vi "SweepCtrlStepCal_DP_ver2.0.vi"(0 "output cluster":T1={"Main Sweep"=0, "Steps Config:"={"total points:"=0, "Step Delay (s)"=0.0, "Ini Delay (s)"=0.0, "# of steps:"=0}, "Temperature Control (ITC 503):"={"GPIB ADR"=0, "Change Heater?"={"Heater?"=FALSE, "Heater"=0}, "Change Temp?"={"Change T?"=FALSE, "Set T (K)"=0.0}, "Cluster"={"Heat Auto?"=FALSE, "Manual Heat?"=FALSE, "Heater (%)"=0.0}, "Change PID?"={"Change PID?"=FALSE, "P"=0.0, "I"=0.0, "D"=0.0}, "Change Para?"=FALSE, "Sensor"=1}, "Temperature Control (LS 340):"={"GPIB ADR"=0, "From (K)"=0.0, "To (K)"=0.0, "Rate (K/min)"=0.0, "Delta T (0.08K)"=0.0, "Temp. Header"="", "T Display Control"={"Ch B"=FALSE, "Ch C"=FALSE, "Ch D"=FALSE}}, "Magnet Control (IPS 120-10)"={"Action"=0, "Standby (s)"=0.0, "Heater on (s)"=0.0, "Sweep Setup "=[], "GPIB ADR"=0, "Change Para?"=FALSE}, "Keithley 6221 :"=[], "Measuring Instruments : "=[], "Lock-In SR7265 :"=[], "Deascription of \nthis measurement"="", "Instruments Config:"=[], "LS372 Bridge : 2"=[{"GPIB"=0, "Excitation"=0, "Autorange?"=FALSE, "Range"=0, "Current"=0, "Voltage"=0, "DataHeader"="Rx;Ry"}], "Magnet Control (CS4) 2"={"Action"=1, "Standby (s)"=0.0, "Heater on (s)"=300.0, "Sweep Setup "=[], "GPIB ADR"=0, "Change Para?"=FALSE}} {"Magnet Control (CS4) 2"."GPIB ADR" items=["None"=0, "25"=25]; "Magnet Control (CS4) 2"."Sweep Setup"."Rate in Range (T/min)" min=0.001 max=0.5 step=0.001; "Magnet Control (CS4) 2"."Sweep Setup"."Hold(min)" min=0.0; "Magnet Control (CS4) 2"."Sweep Setup"."Set Point (T)" min=-9.0 max=9.0 step=0.001; "Magnet Control (CS4) 2"."Action" items=["Up", "Down", "Pause", "Zero"]; "LS372 Bridge : 2"."Voltage" items=["2.00 uV"=1, "6.32 uV"=2, "20.0 uV"=3, "63.2 uV"=4, "200 uV"=5, "632 uV"=6, "2.0 mV"=7, "6.32 mV"=8]; "LS372 Bridge : 2"."Current" items=["1.00 pA"=1, "3.16 pA"=2, "10.0 pA"=3, "31.6 pA"=4, "100 pA"=5, "316 pA"=6, "1.00 nA"=7, "3.16 nA"=8, "10 nA"=9, "31.6 nA"=10, "100 nA"=11, "316 nA"=12, "1.00 uA"=13, "3.16 uA"=14, "10.0 uA"=15, "31.6 uA"=16, "100 uA"=17, "316 uA"=18, "1.00 mA"=19, "3.16 mA"=20, "10.0 mA"=21, "31.6 mA"=22]; "LS372 Bridge : 2"."Range" items=["2.0 m"=1, "6.32 m"=2, "20.0 m"=3, "63.2 m"=4, "200 m"=5, "632 m"=6, "2.00"=7, "6.32"=8, "20.0"=9, "63.2"=10, "200"=11, "632"=12, "2.00 k"=13, "6.32 k"=14, "20.0 k"=15, "63.2 k"=16, "200 k"=17, "632 k"=18, "2.00 M"=19, "6.32 M"=20, "20.0 M"=21, "63.2 M"=22]; "LS372 Bridge : 2"."Excitation" items=["Voltage", "Current"]; "LS372 Bridge : 2"."GPIB" items=["None"=0, "9"=9]; "Main Sweep" items=["Time", "DC Current", "Delta Current", "Pulse Delta Current", "Sine Current", "Lock-in Vosc"]; "Temperature Control (ITC 503):"."Sensor" items=["T2", "T3"]; "Magnet Control (IPS 120-10)"."Action" items=["Hold", "To Set point", "To Zero", "Clamp"]; "Keithley 6221 :"."Sweep Mode" items=["Linear", "Log", "Exp", "Inverse", "Manual"]}) -> (1 "Stay duration pts":dbl[](array[numeric]), 2 "2D Array of DC Source or Lock-In Ctrl Run Cluster":cluster{"GPIB ADR":u16, "DC St. Pt.":dbl}[][](array[cluster]))   [LabVIEW 2012]
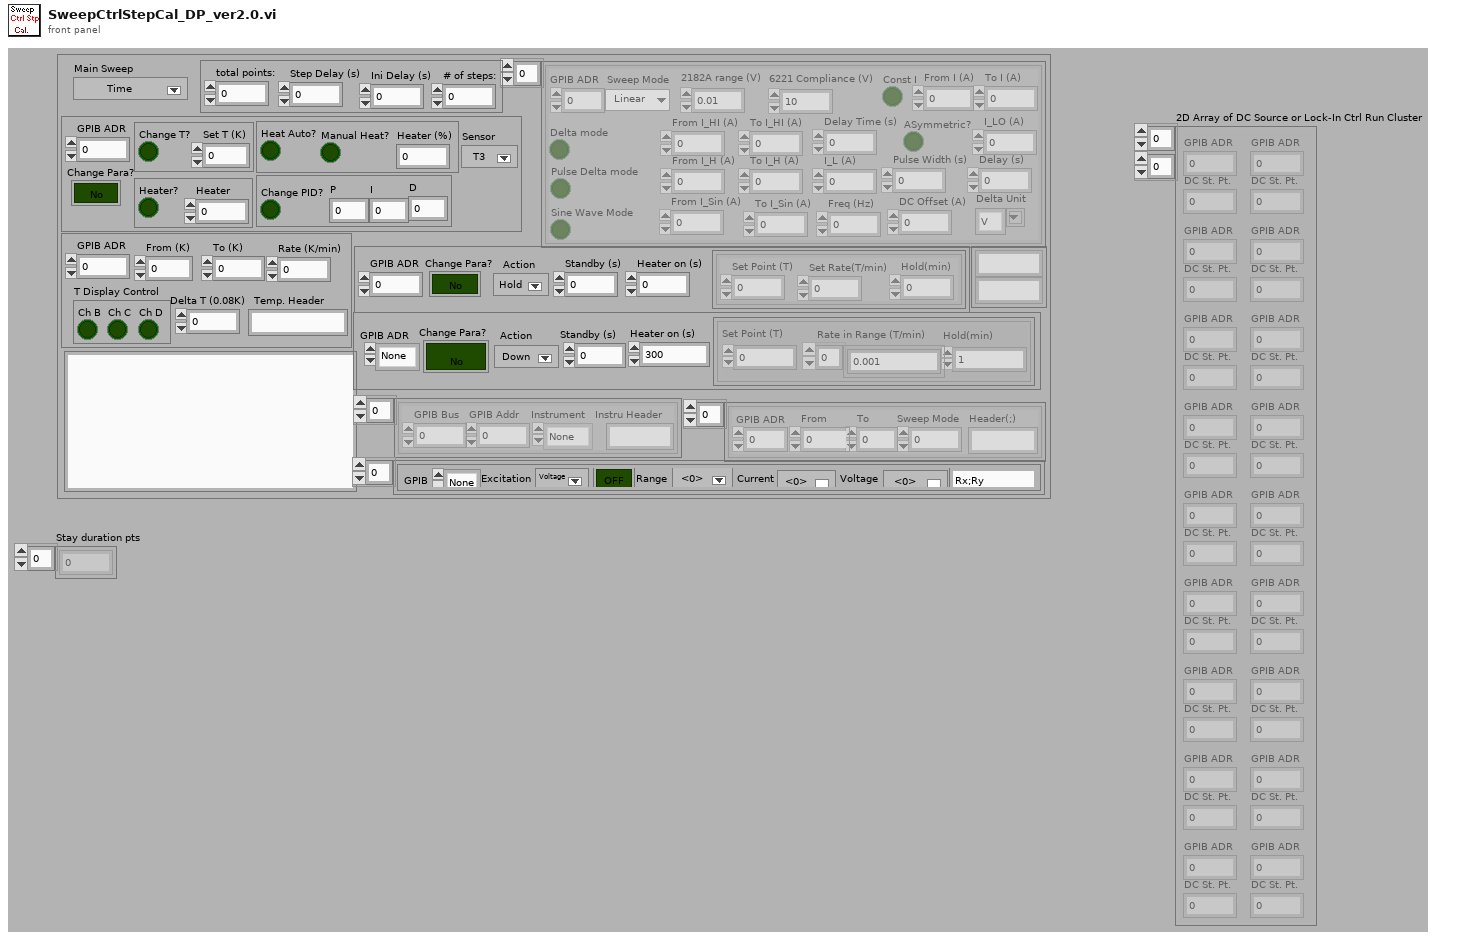
[diagram p1: front panel]
types:
  T1 = cluster{"Main Sweep":u8, "Steps Config:":cluster{"total points:":u32, "Step Delay (s)":dbl, "Ini Delay (s)":dbl, "# of steps:":u32}, "Temperature Control (ITC 503):":cluster{"GPIB ADR":u16, "Change Heater?":cluster{"Heater?":bool, "Heater":u8}, "Change Temp?":cluster{"Change T?":bool, "Set T (K)":dbl}, "Cluster":cluster{"Heat Auto?":bool, "Manual Heat?":bool, "Heater (%)":dbl}, "Change PID?":cluster{"Change PID?":bool, "P":dbl, "I":dbl, "D":dbl}, "Change Para?":bool, "Sensor":u16}, "Temperature Control (LS 340):":cluster{"GPIB ADR":u16, "From (K)":dbl, "To (K)":dbl, "Rate (K/min)":dbl, "Delta T (0.08K)":dbl, "Temp. Header":string, "T Display Control":cluster{"Ch B":bool, "Ch C":bool, "Ch D":bool}}, "Magnet Control (IPS 120-10)":cluster{"Action":u16, "Standby (s)":dbl, "Heater on (s)":dbl, "Sweep Setup ":cluster{"Set Point (T)":dbl, "Set Rate(T/min)":dbl, "Hold(min)":dbl}[], "GPIB ADR":u16, "Change Para?":bool}, "Keithley 6221 :":cluster{"Delta mode":bool, "Const I":bool, "Pulse Delta mode":bool, "Sine Wave Mode":bool, "From I_HI (A)":dbl, "From I (A)":dbl, "I_LO (A)":dbl, "From I_H (A)":dbl, "I_L (A)":dbl, "Freq (Hz)":dbl, "From I_Sin (A)":dbl, "DC Offset (A)":dbl, "Delay Time (s)":dbl, "Pulse Width (s)":dbl, "Delay (s)":dbl, "To I (A)":dbl, "ASymmetric?":bool, "To I_HI (A)":dbl, "To I_H (A)":dbl, "To I_Sin (A)":dbl, "GPIB ADR":u16, "Sweep Mode":u8, "Delta Unit":string, "2182A range (V)":dbl, "6221 Compliance (V)":dbl}[], "Measuring Instruments : ":cluster{"GPIB Bus":dbl, "GPIB Addr":dbl, "Instrument":enum16{"None", "HP34401DMM", "Lockin 7265", "HP3456/7A", "HP3478A", "HP3325FG", "Keithley2182A"}, "Instru Header":string}[], "Lock-In SR7265 :":cluster{"GPIB ADR":u16, "From":dbl, "To":dbl, "Header(;)":string, "Sweep Mode":u8}[], "Deascription of \nthis measurement":string, "Instruments Config:":string[][], "LS372 Bridge : 2":cluster{"GPIB":u16, "Excitation":u16, "Autorange?":bool, "Range":u16, "Current":u16, "Voltage":u16, "DataHeader":string}[], "Magnet Control (CS4) 2":cluster{"Action":u16, "Standby (s)":dbl, "Heater on (s)":dbl, "Sweep Setup ":cluster{"Set Point (T)":dbl, "Hold(min)":dbl, "Rate in Range (T/min)":dbl[]}[], "GPIB ADR":u16, "Change Para?":bool}}
  T2 = cluster{"total points:":u32, "Step Delay (s)":dbl, "Ini Delay (s)":dbl, "# of steps:":u32}
  T3 = cluster{"GPIB ADR":u16, "From":dbl, "To":dbl, "Header(;)":string, "Sweep Mode":u8}[]
  T4 = cluster{"Delta mode":bool, "Const I":bool, "Pulse Delta mode":bool, "Sine Wave Mode":bool, "From I_HI (A)":dbl, "From I (A)":dbl, "I_LO (A)":dbl, "From I_H (A)":dbl, "I_L (A)":dbl, "Freq (Hz)":dbl, "From I_Sin (A)":dbl, "DC Offset (A)":dbl, "Delay Time (s)":dbl, "Pulse Width (s)":dbl, "Delay (s)":dbl, "To I (A)":dbl, "ASymmetric?":bool, "To I_HI (A)":dbl, "To I_H (A)":dbl, "To I_Sin (A)":dbl, "GPIB ADR":u16, "Sweep Mode":u8, "Delta Unit":string, "2182A range (V)":dbl, "6221 Compliance (V)":dbl}[]
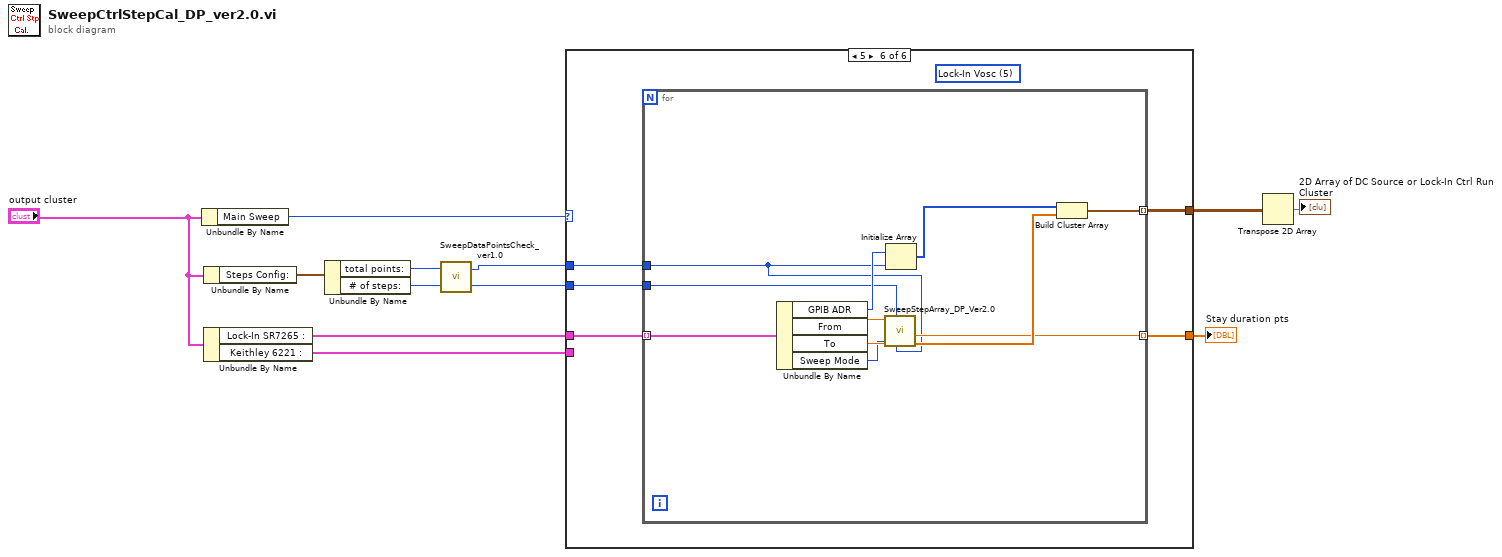
[diagram p0: block diagram]
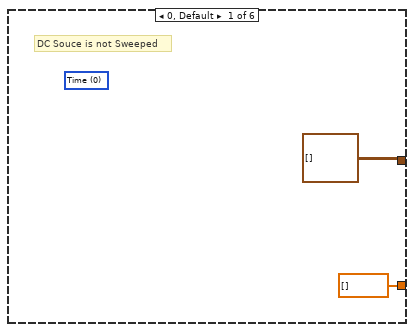
[diagram p2: hidden frame]
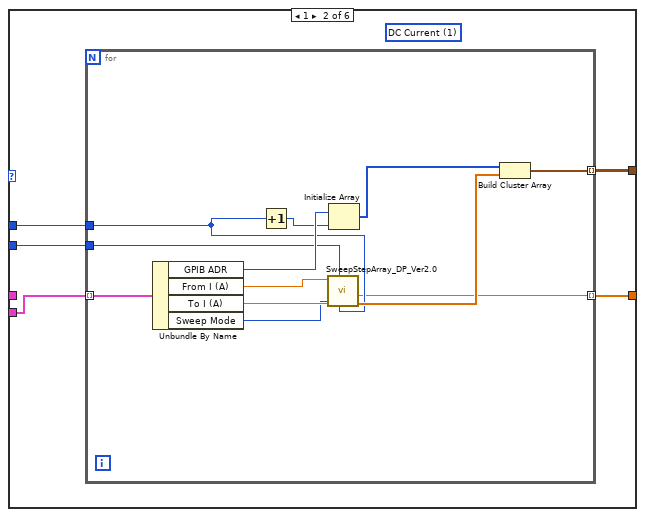
[diagram p3: hidden frame]
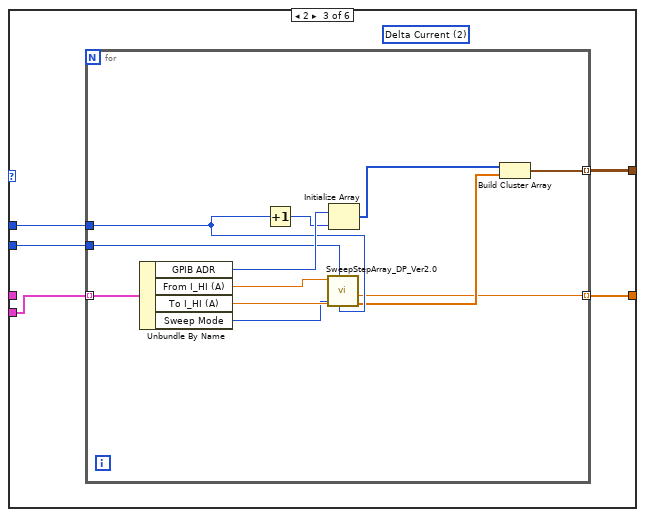
[diagram p4: hidden frame]
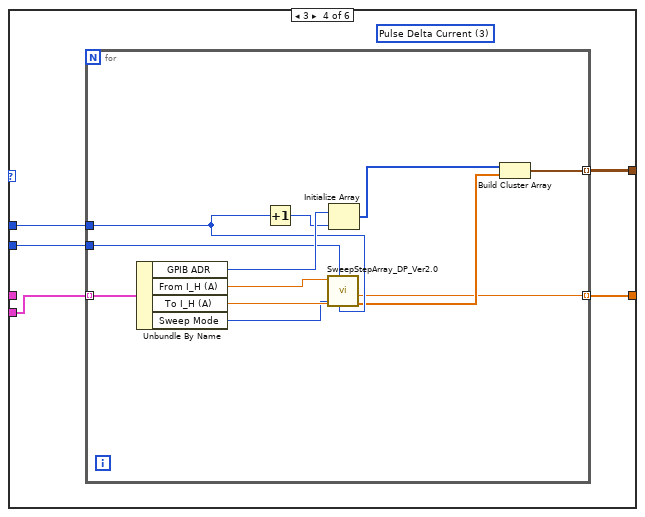
[diagram p5: hidden frame]
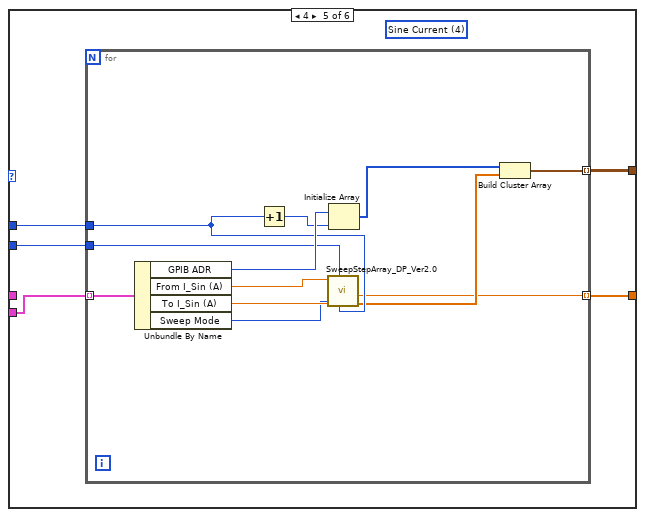
[diagram p6: hidden frame]
diagram:
  n1 = Unbundle By Name("output cluster") -> ("Main Sweep"=w10:u8)
  n2 = Unbundle By Name("output cluster") -> ("Steps Config:"=w9:T2)
  n3 = Unbundle By Name("output cluster") -> ("Lock-In SR7265 :"=w11:T3, "Keithley 6221 :"=w8:T4)
  n4 = Unbundle By Name(w9) -> ("total points:"=w7:u32, "# of steps:"=w6:u32)
  n5 = call "SweepDataPointsCheck_ver1.0.vi"("Input # of sweep steps:"=w6, "Input # of total points:"=w7) -> ("Output # of sweep steps:"=w2:u32, "Output # of total points:"=w5:u32)
  n6 = case shown="5" w10 {
    tunnel: [cluster{"GPIB ADR":u16, "V Start":dbl}[][] [] ("array of clusters") w19 w36 w53 w70 w87] -> w4
    tunnel: w11 -> [_ _ _ _ _ w86]
    tunnel: w5 -> [_ w18 w35 w52 w69 w85]
    tunnel: w2 -> [_ w17 w34 w51 w68 w84]
    tunnel: w8 -> [_ w16 w33 w50 w67 _]
    tunnel: [dbl[] [] w15 w32 w49 w66 w83] -> w3
    frame 0, Default {
      (unwired) u8 0 items=["Time", "DC Current", "Delta Current", "Pulse Delta Current", "Sine Current", "Lock-In Vosc"] ("Main Sweep")
      # "DC Souce is not Sweeped"
    }
    frame 1 {
      (unwired) u8 1 items=["Time", "DC Current", "Delta Current", "Pulse Delta Current", "Sine Current", "Lock-In Vosc"] ("Main Sweep")
      n7 = for {
        tunnel: w16 -> [w31] mode=indexing
        tunnel: [w21] -> w19 mode=indexing
        tunnel: w18 -> [w23]
        tunnel: w17 -> [w26]
        tunnel: [w20] -> w15 mode=indexing
        n8 = Unbundle By Name(w31) -> ("GPIB ADR"=w27:u16, "From I (A)"=w30:dbl, "To I (A)"=w29:dbl, "Sweep Mode"=w28:u8)
        n9 = Increment(x=w23) -> (x+1=w22:u32)
        n10 = call "SweepStepArray_DP_Ver2.0.vi"("# of total points:"=w23, "# of sweep steps:"=w26, "Sweep Mode"=w28, "Stop"=w29, "Start"=w30) -> ("Array Out"=w25:dbl[], "Stay duration points"=w20:dbl)  [unwired: 2 in, 1 out]
        n11 = Initialize Array(w27, w22) -> (w24:u16[])
        n12 = Build Cluster Array(w24, w25) -> (w21:cluster{"GPIB ADR":u16, "V Start":dbl}[])
      }
    }
    frame 2 {
      (unwired) u8 2 items=["Time", "DC Current", "Delta Current", "Pulse Delta Current", "Sine Current", "Lock-In Vosc"] ("Main Sweep")
      n13 = for {
        tunnel: w33 -> [w48] mode=indexing
        tunnel: [w39] -> w36 mode=indexing
        tunnel: w35 -> [w43]
        tunnel: w34 -> [w42]
        tunnel: [w37] -> w32 mode=indexing
        n14 = Unbundle By Name(w48) -> ("GPIB ADR"=w44:u16, "From I_HI (A)"=w47:dbl, "To I_HI (A)"=w46:dbl, "Sweep Mode"=w45:u8)
        n15 = Increment(x=w43) -> (x+1=w38:u32)
        n16 = call "SweepStepArray_DP_Ver2.0.vi"("# of total points:"=w43, "# of sweep steps:"=w42, "Sweep Mode"=w45, "Stop"=w46, "Start"=w47) -> ("Array Out"=w41:dbl[], "Stay duration points"=w37:dbl)  [unwired: 2 in, 1 out]
        n17 = Initialize Array(w44, w38) -> (w40:u16[])
        n18 = Build Cluster Array(w40, w41) -> (w39:cluster{"GPIB ADR":u16, "V Start":dbl}[])
      }
    }
    frame 3 {
      (unwired) u8 3 items=["Time", "DC Current", "Delta Current", "Pulse Delta Current", "Sine Current", "Lock-In Vosc"] ("Main Sweep")
      n19 = for {
        tunnel: w50 -> [w65] mode=indexing
        tunnel: [w56] -> w53 mode=indexing
        tunnel: w52 -> [w60]
        tunnel: w51 -> [w59]
        tunnel: [w54] -> w49 mode=indexing
        n20 = Unbundle By Name(w65) -> ("GPIB ADR"=w61:u16, "From I_H (A)"=w64:dbl, "To I_H (A)"=w63:dbl, "Sweep Mode"=w62:u8)
        n21 = Increment(x=w60) -> (x+1=w55:u32)
        n22 = call "SweepStepArray_DP_Ver2.0.vi"("# of total points:"=w60, "# of sweep steps:"=w59, "Sweep Mode"=w62, "Stop"=w63, "Start"=w64) -> ("Array Out"=w58:dbl[], "Stay duration points"=w54:dbl)  [unwired: 2 in, 1 out]
        n23 = Initialize Array(w61, w55) -> (w57:u16[])
        n24 = Build Cluster Array(w57, w58) -> (w56:cluster{"GPIB ADR":u16, "V Start":dbl}[])
      }
    }
    frame 4 {
      (unwired) u8 4 items=["Time", "DC Current", "Delta Current", "Pulse Delta Current", "Sine Current", "Lock-In Vosc"] ("Main Sweep")
      n25 = for {
        tunnel: w67 -> [w82] mode=indexing
        tunnel: [w73] -> w70 mode=indexing
        tunnel: w69 -> [w77]
        tunnel: w68 -> [w76]
        tunnel: [w71] -> w66 mode=indexing
        n26 = Unbundle By Name(w82) -> ("GPIB ADR"=w78:u16, "From I_Sin (A)"=w81:dbl, "To I_Sin (A)"=w80:dbl, "Sweep Mode"=w79:u8)
        n27 = Increment(x=w77) -> (x+1=w72:u32)
        n28 = call "SweepStepArray_DP_Ver2.0.vi"("# of total points:"=w77, "# of sweep steps:"=w76, "Sweep Mode"=w79, "Stop"=w80, "Start"=w81) -> ("Array Out"=w75:dbl[], "Stay duration points"=w71:dbl)  [unwired: 2 in, 1 out]
        n29 = Initialize Array(w78, w72) -> (w74:u16[])
        n30 = Build Cluster Array(w74, w75) -> (w73:cluster{"GPIB ADR":u16, "V Start":dbl}[])
      }
    }
    frame 5 {
      (unwired) u8 5 items=["Time", "DC Current", "Delta Current", "Pulse Delta Current", "Sine Current", "Lock-In Vosc"] ("Main Sweep")
      n31 = for {
        tunnel: w86 -> [w98] mode=indexing
        tunnel: [w90] -> w87 mode=indexing
        tunnel: w85 -> [w88]
        tunnel: w84 -> [w93]
        tunnel: [w89] -> w83 mode=indexing
        n32 = Unbundle By Name(w98) -> ("GPIB ADR"=w94:u16, "From"=w97:dbl, "To"=w96:dbl, "Sweep Mode"=w95:u8)
        n33 = call "SweepStepArray_DP_Ver2.0.vi"("# of total points:"=w88, "# of sweep steps:"=w93, "Sweep Mode"=w95, "Stop"=w96, "Start"=w97) -> ("Array Out"=w92:dbl[], "Stay duration points"=w89:dbl)  [unwired: 2 in, 1 out]
        n34 = Initialize Array(w94, w88) -> (w91:u16[])
        n35 = Build Cluster Array(w91, w92) -> (w90:cluster{"GPIB ADR":u16, "V Start":dbl}[])
      }
    }
  }
  "Stay duration pts" <- w3
  n36 = Transpose 2D Array(2D array=w4) -> (transposed array=→"2D Array of DC Source or Lock-In Ctrl Run Cluster":cluster{"GPIB ADR":u16, "V Start":dbl}[][])
